vi "Action Name.vi"(8 "error in (no error)":errorcluster, 11 "Filter by Is Action In":refnum<class "Filter by Is Action.lvclass">) -> (0 "error out":errorcluster, 2 "Action Name":string, 3 "Filter by Is Action Out":refnum<class "Filter by Is Action.lvclass">)   [LabVIEW 2020, in "Filter by Is Action.lvclass"]
uses:
  Filter by Is Action.lvclass
  Filter by Is Action.lvclass/Filter by Is Action.ctl
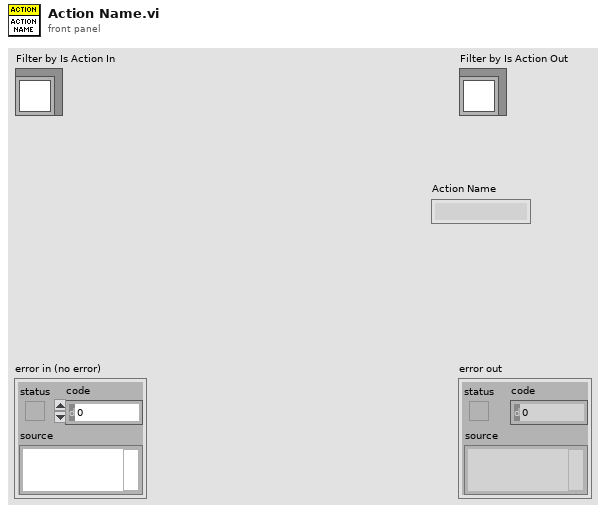
[diagram p1: front panel]
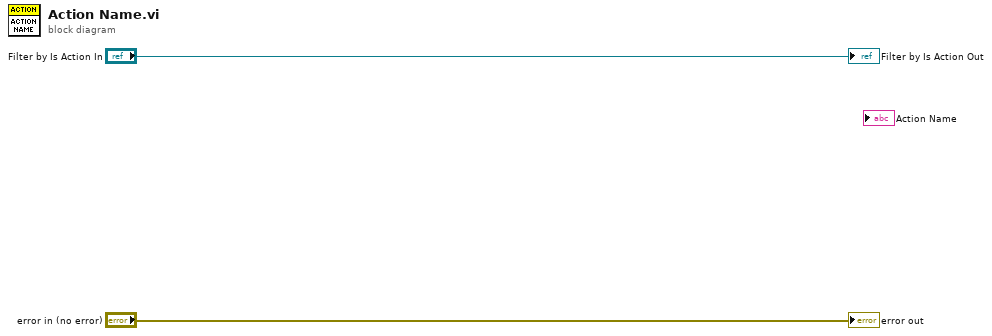
[diagram p0: block diagram]
diagram:
  "error out" <- "error in (no error)"
  "Filter by Is Action Out" <- "Filter by Is Action In"
